vi "Easy2Acquire.IDevice.Acquire.Simple.vi"(0 "IDeviceIn":refnum<k7>, 1 "IAnalogInput":refnum<k7>[](array[refnum]), 3 "DigitalInput":refnum<k7>[](array[refnum]), 4 "MotionInput":refnum<k7>[](array[refnum]), 5 "error in (no error)":errorcluster) -> (14 "AnalogBuffer":dbl[][](array[numeric]), 17 "MotionBuffer":dbl[][][](array[numeric]), 18 "Euler":dbl[][](array[numeric]), 19 "error out":errorcluster)   [LabVIEW 2015]
panel:
  out "DigitalFrequency":dbl[](array[numeric])
  out "MotionFrequency":dbl[](array[numeric])
  out "DigitalBuffer":i32[][](array[numeric])
  out "ActualFrequency":dbl[](array[numeric])
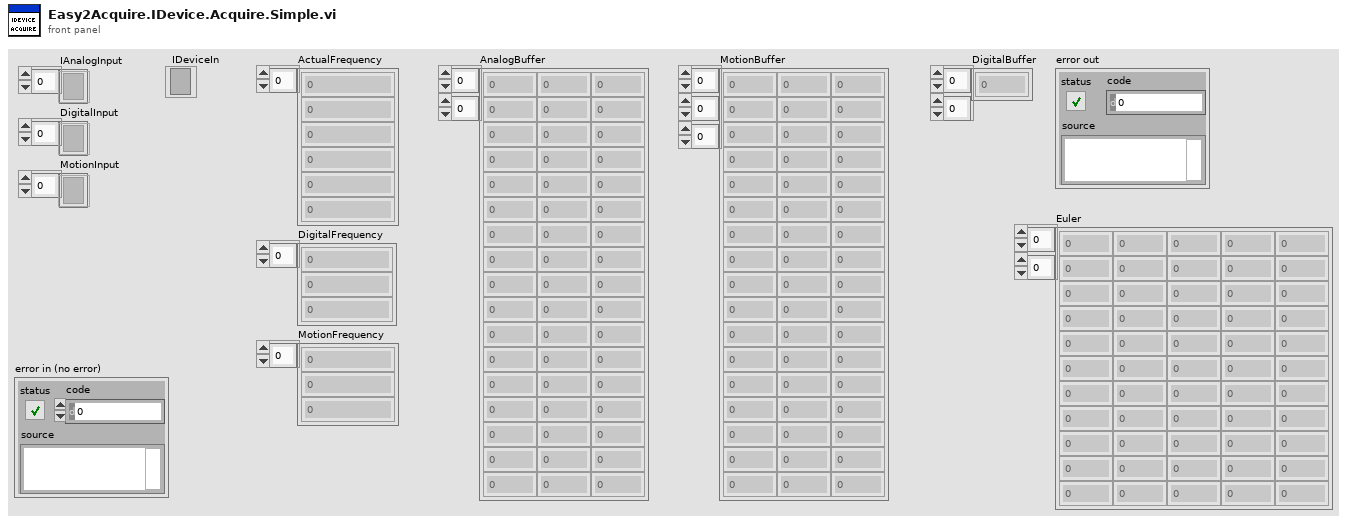
[diagram p1: front panel]
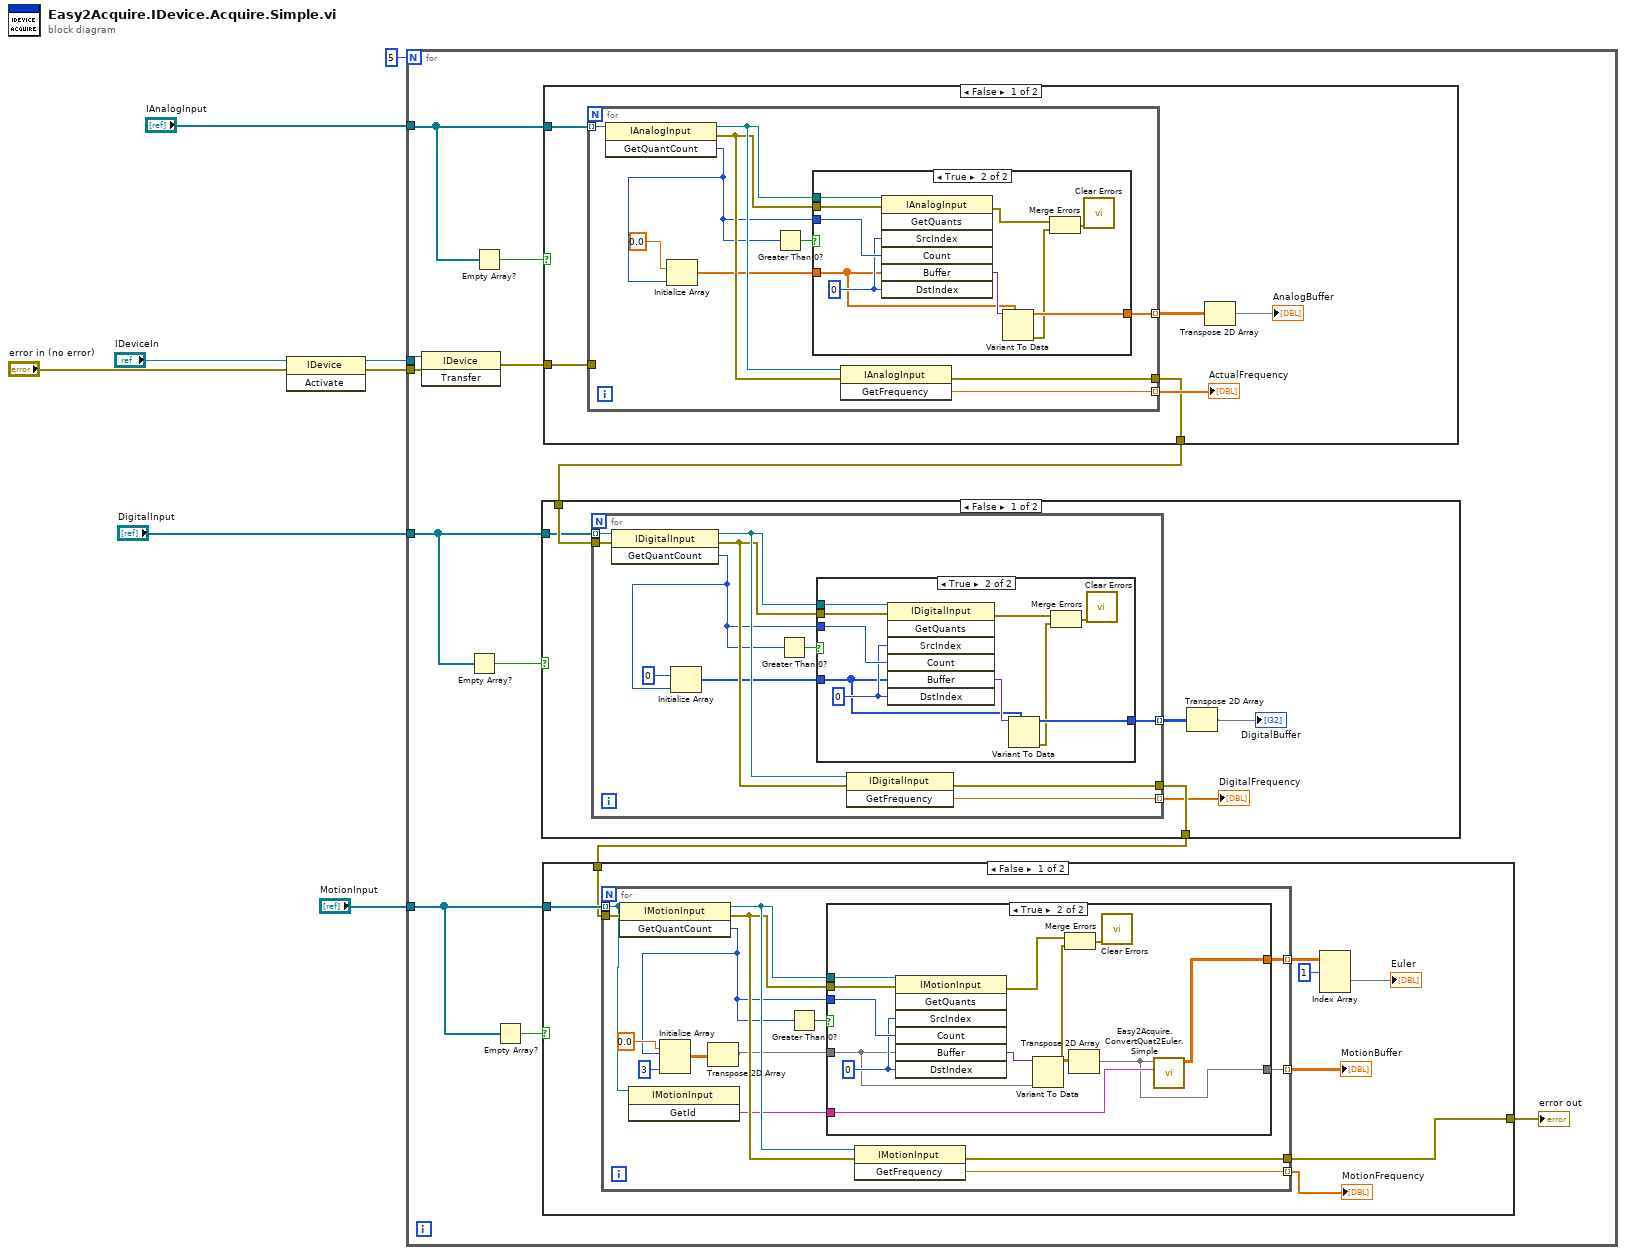
[diagram p0: block diagram]
diagram:
  n1 = invoke class="IDevice" method="Activate"(reference="IDeviceIn", error in="error in (no error)") -> (reference out=w7:refnum<k7>, error out=w6:errorcluster)  [unwired: 1 in, 1 out]
  n2 = for {
    N: 5 -> [_]
    tunnel: "IAnalogInput" -> [w20]
    tunnel: w7 -> [w19]
    tunnel: w6 -> [w18]
    tunnel: "DigitalInput" -> [w17]
    tunnel: "MotionInput" -> [w16]
    n3 = invoke class="IDevice" method="Transfer"(reference=w19, error in=w18) -> (error out=w14:errorcluster)  [unwired: 1 in, 2 out]
    n4 = Empty Array?(array=w17) -> (empty?=w10:bool)
    n5 = Empty Array?(array=w20) -> (empty?=w11:bool)
    n6 = Empty Array?(array=w16) -> (empty?=w9:bool)
    n7 = case shown="False" w11 {
      tunnel: w20 -> [w91 _]
      tunnel: w14 -> [w89 w112]
      tunnel: [w88 w112] -> w13
      frame False {
        n8 = for {
          tunnel: w91 -> [w101] mode=indexing
          tunnel: [w99] -> w90 mode=indexing
          tunnel: [w93] -> w87 mode=indexing
          tunnel: w89 -> [_]
          tunnel: [w92] -> w88
          n9 = invoke class="IAnalogInput" method="GetQuantCount"(reference=w101) -> (reference out=w98:refnum<k7>, error out=w97:errorcluster, "GetQuantCount"=w95:i32)  [unwired: 2 in]
          n10 = Initialize Array(0.0, w95) -> (w96:dbl[])
          n11 = Greater Than 0?(x=w95) -> (x > 0?=w100:bool)
          n12 = case shown="True" w100 {
            tunnel: w98 -> [_ w111]
            tunnel: w95 -> [_ w110]
            tunnel: w97 -> [_ w108]
            tunnel: w96 -> [_ w106]
            tunnel: [_ w105] -> w93
            frame False {
            }
            frame True {
              w109 = 0 ("SrcIndex")
              n13 = invoke class="IAnalogInput" method="GetQuants"(reference=w111, error in=w108, "SrcIndex"=w109, "Count"=w110, "Buffer"=w106, "DstIndex"=w109) -> (error out=w103:errorcluster, "Buffer"=w107:variant)  [unwired: 1 in, 5 out]
              n14 = Variant To Data(type=w106, Variant=w107) -> (data=w105:dbl[], error out=w102:errorcluster)  [unwired: 1 in]
              n15 = Merge Errors(w103, w102) -> (w104:errorcluster)
              n16 = call <vilib>:"Clear Errors.vi"("error in (no error)"=w104) -> ()  [unwired: 5 in, 2 out]
            }
          }
          n17 = invoke class="IAnalogInput" method="GetFrequency"(reference=w98, error in=w97) -> (error out=w92:errorcluster, "GetFrequency"=w99:dbl)  [unwired: 1 in, 1 out]
        }
        "ActualFrequency" <- w90
        n18 = Transpose 2D Array(2D array=w87) -> (transposed array=→"AnalogBuffer":dbl[][])
      }
      frame True {
      }
    }
    n19 = case shown="False" w10 {
      tunnel: w13 -> [w63 w85]
      tunnel: w17 -> [w62 _]
      tunnel: [w61 w85] -> w12
      frame False {
        n20 = for {
          tunnel: [w73] -> w58 mode=indexing
          tunnel: [w68] -> w60 mode=indexing
          tunnel: w63 -> [w67]
          tunnel: w62 -> [w66] mode=indexing
          tunnel: [w65] -> w61
          n21 = invoke class="IDigitalInput" method="GetQuantCount"(reference=w66, error in=w67) -> (reference out=w72:refnum<k7>, error out=w71:errorcluster, "GetQuantCount"=w69:i32)  [unwired: 1 in]
          n22 = Initialize Array(u8 0, w69) -> (w70:u8[])
          n23 = Greater Than 0?(x=w69) -> (x > 0?=w74:bool)
          n24 = case shown="True" w74 {
            tunnel: w72 -> [_ w84]
            tunnel: w69 -> [_ w83]
            tunnel: w71 -> [_ w81]
            tunnel: w70 -> [_ w79]
            tunnel: [_ w78] -> w68
            frame False {
            }
            frame True {
              w82 = 0 ("SrcIndex")
              n25 = invoke class="IDigitalInput" method="GetQuants"(reference=w84, error in=w81, "SrcIndex"=w82, "Count"=w83, "Buffer"=w79, "DstIndex"=w82) -> (error out=w76:errorcluster, "Buffer"=w80:variant)  [unwired: 1 in, 5 out]
              n26 = Variant To Data(type=w79, Variant=w80) -> (data=w78:u8[], error out=w75:errorcluster)  [unwired: 1 in]
              n27 = Merge Errors(w76, w75) -> (w77:errorcluster)
              n28 = call <vilib>:"Clear Errors.vi"("error in (no error)"=w77) -> ()  [unwired: 5 in, 2 out]
            }
          }
          n29 = invoke class="IDigitalInput" method="GetFrequency"(reference=w72, error in=w71) -> (error out=w65:errorcluster, "GetFrequency"=w73:dbl)  [unwired: 1 in, 1 out]
        }
        "DigitalFrequency" <- w58
        n30 = Transpose 2D Array(2D array=w60) -> (transposed array=→"DigitalBuffer":u8[][])
      }
      frame True {
      }
    }
    n31 = case shown="False" w9 {
      tunnel: w16 -> [w28 _]
      tunnel: w12 -> [w26 w57]
      tunnel: [w25 w57] -> w15
      frame False {
        n32 = for {
          tunnel: w28 -> [w31] mode=indexing
          tunnel: [w42] -> w24 mode=indexing
          tunnel: [w38] -> w27 mode=indexing
          tunnel: w26 -> [w37]
          tunnel: [w36] -> w25
          tunnel: [w29] -> w23 mode=indexing
          n33 = invoke class="IMotionInput" method="GetQuantCount"(reference=w31, error in=w37) -> (reference out=w41:refnum<k7>, error out=w40:errorcluster, "GetQuantCount"=w35:i32)  [unwired: 1 in]
          n34 = invoke class="IMotionInput" method="GetId"(reference=w31) -> ("GetId"=w30:string)  [unwired: 2 in, 2 out]
          n35 = Initialize Array(0.0, w35, 3 ("dimension size")) -> (w33:dbl[][])
          n36 = Transpose 2D Array(2D array=w33) -> (transposed array=w32:dbl[][])
          n37 = Greater Than 0?(x=w35) -> (x > 0?=w43:bool)
          n38 = case shown="True" w43 {
            tunnel: w41 -> [_ w56]
            tunnel: w35 -> [_ w55]
            tunnel: w40 -> [_ w53]
            tunnel: w32 -> [_ w51]
            tunnel: [_ w45] -> w38
            tunnel: w30 -> [_ w46]
            tunnel: [_ w44] -> w29
            frame False {
            }
            frame True {
              w54 = 0 ("SrcIndex")
              n39 = invoke class="IMotionInput" method="GetQuants"(reference=w56, error in=w53, "SrcIndex"=w54, "Count"=w55, "Buffer"=w51, "DstIndex"=w54) -> (error out=w49:errorcluster, "Buffer"=w52:variant)  [unwired: 1 in, 5 out]
              n40 = Variant To Data(type=w51, Variant=w52) -> (data=w47:dbl[][], error out=w50:errorcluster)  [unwired: 1 in]
              n41 = Merge Errors(w49, w50) -> (w48:errorcluster)
              n42 = Transpose 2D Array(2D array=w47) -> (transposed array=w45:dbl[][])
              n43 = call <vilib>:"Clear Errors.vi"("error in (no error)"=w48) -> ()  [unwired: 5 in, 2 out]
              n44 = call "Easy2Acquire.ConvertQuat2Euler.Simple.vi"("GetID"=w46, "MotionData"=w45) -> ("Accel"=w44:dbl[][])  [unwired: 8 in, 1 out]
            }
          }
          n45 = invoke class="IMotionInput" method="GetFrequency"(reference=w41, error in=w40) -> (error out=w36:errorcluster, "GetFrequency"=w42:dbl)  [unwired: 1 in, 1 out]
        }
        "MotionBuffer" <- w27
        "MotionFrequency" <- w24
        n46 = Index Array(array=w23, index (dim 0)=1 ("index (page)")) -> (element=→"Euler":dbl[][])  [unwired: 2 in]
      }
      frame True {
      }
    }
    "error out" <- w15
  }
